vi "NI6008 Status Report.vi"(8 "error in (no error)":errorcluster, 10 "Data":T1, 11 "Controller in":refnum<class "Controller.lvclass">) -> (0 "error out":errorcluster, 3 "Controller out":refnum<class "Controller.lvclass">)   [LabVIEW 2020, in "Controller.lvlib" / "Controller.lvclass"]
uses:
  Controller.lvclass
  C:/Program Files/National Instruments/LabVIEW 2020/vi.lib/ActorFramework/Actor/Actor.lvclass
  <vilib>/ActorFramework/Actor/Actor.lvclass/Actor.ctl
  <vilib>/ActorFramework/Message Enqueuer/Message Enqueuer.lvclass/Message Enqueuer.ctl
  Controller.lvclass/Controller.ctl
  Actor_log/Actor_log Messages/Write Event to Log Msg/Write Event to Log Msg.lvclass/Write Event to Log Msg.ctl
  <vilib>/ActorFramework/Message Enqueuer/Init from Existing Queue.vi
  <vilib>/ActorFramework/Message Enqueuer/Enqueue.vi
  <vilib>/ActorFramework/Stop Msg/Send Emergency Stop.vi
  <vilib>/ActorFramework/Stop Msg/Send Normal Stop.vi
  <vilib>/ActorFramework/Message Enqueuer/Enqueue Critical.vi
  Actor_log/Actor_log Messages/Write Event to Log Msg/Write Event to Log Msg.lvclass
  C:/Program Files/National Instruments/LabVIEW 2020/vi.lib/ActorFramework/Message/Message.lvclass
  <vilib>/ActorFramework/Stop Msg/Stop Msg.lvclass
  <vilib>/ActorFramework/Message Priority Queue/Priority Enqueue.vi
  <vilib>/ActorFramework/Message Enqueuer/Message Enqueuer.lvclass
  <vilib>/ActorFramework/Actor/Actor.lvclass
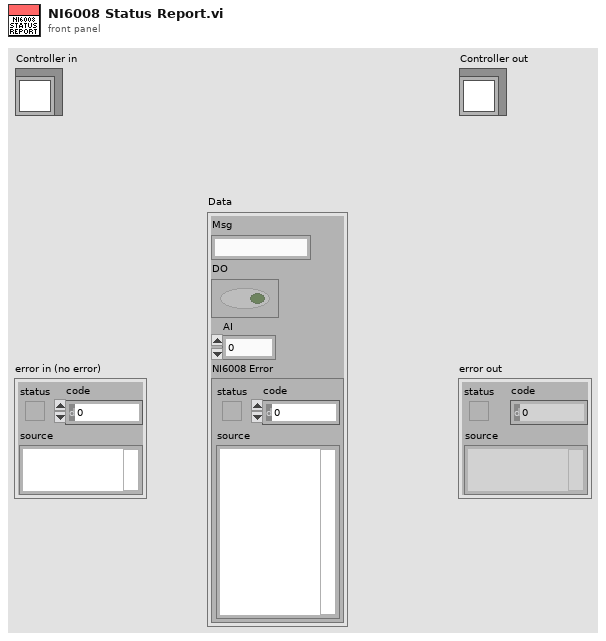
[diagram p1: front panel]
types:
  T1 = cluster{"Msg":string, "DO":bool[], "AI":dbl, "NI6008 Error":errorcluster}
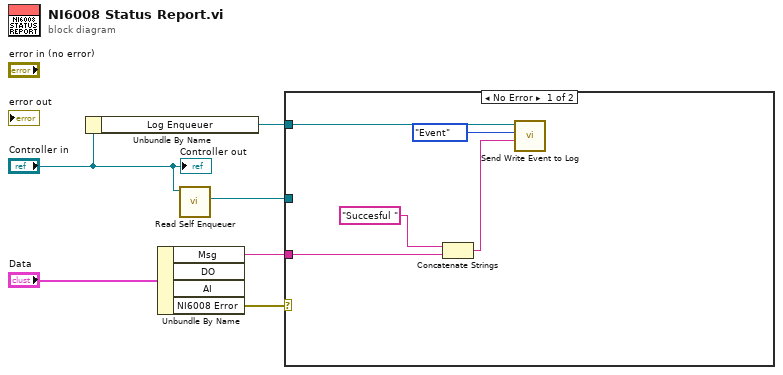
[diagram p0: block diagram]
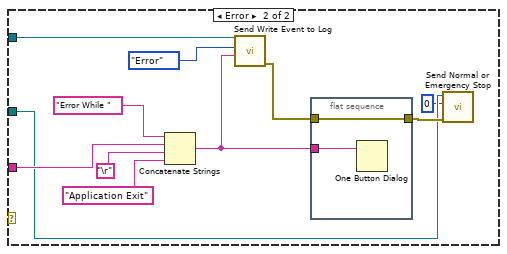
[diagram p2: hidden frame]
diagram:
  n1 = Unbundle By Name("Controller in") -> ("Log Enqueuer"=w3:refnum<class "Message Enqueuer.lvclass">)
  n2 = Unbundle By Name("Data") -> ("Msg"=w4:string, "NI6008 Error"=w5:errorcluster)  [unwired: 2 out]
  n3 = call <vilib>:"Read Self Enqueuer.vi"("Actor"="Controller in") -> ("Self Enqueuer"=w1:refnum<class "Message Enqueuer.lvclass">)  [unwired: 10 in]
  n4 = case shown="No Error" w5 {
    tunnel: w4 -> [w9 w18]
    tunnel: w3 -> [w11 w19]
    tunnel: w1 -> [_ w13]
    frame No Error {
      n5 = Concatenate Strings("Succesful " ("string"), w9) -> (w7:string)
      n6 = call "Send Write Event to Log.vi"("Log Event Details"=w7, "Enum"=enum16{"Event", "Error"}."Event", "Message Enqueuer"=w11) -> ()  [unwired: 7 in, 2 out]
    }
    frame Error {
      n7 = Concatenate Strings("Error While " ("string"), w18, "\r", "Application Exit" ("string")) -> (w15:string)
      n8 = call "Send Write Event to Log.vi"("Log Event Details"=w15, "Enum"=enum16{"Event", "Error"}."Error", "Message Enqueuer"=w19) -> ("error out"=w16:errorcluster)  [unwired: 7 in, 1 out]
      n9 = flat-sequence {
        tunnel: w16 -> [w23]
        tunnel: w15 -> [w24]
        tunnel: [w23] -> w14
        frame #0 {
          n10 = One Button Dialog(message=w24) -> ()  [unwired: 1 in, 1 out]
        }
      }
      n11 = call <vilib>:"Send Normal or Emergency Stop.vi"("error in (no error)"=w14, "final error code"=0, "Message Enqueuer"=w13) -> ()  [unwired: 8 in, 1 out]
    }
  }
  "Controller out" <- "Controller in"
